vi "Connect Channels (Multiple).vi"(8 "error in (no error)":errorcluster, 10 "connection list":string, 11 "SLSC Switch in":refnum<class "SLSC Switch.lvclass">) -> (0 "error out":errorcluster, 3 "SLSC Switch out":refnum<class "SLSC Switch.lvclass">)   [LabVIEW 2015, in "SLSC Switch.lvlib" / "SLSC Switch.lvclass"]
doc: "Creates the connections between channels specified in connection list. Specify connections with two endpoints only or the explicit path between two endpoints. SLSC-SWITCH calculates and uses the shortest path between the channels. Refer to Setting Source and Configuration Channels for information about channel usage types. In the event of an error, connecting stops at the point in the list where the error occurred."
uses:
  SLSC Switch.lvclass
  slscsl/slscsl.lvclass
  <vilib>/SLSC/SLSC.lvlib
  <vilib>/SLSC/Unflatten Names (String).vi
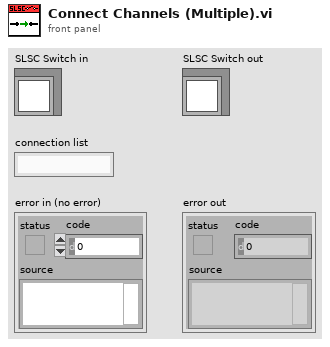
[diagram p1: front panel]
types:
  T1 = typedef "SLSC Switch.lvlib/slscsl.lvclass/SwitchActionsArray.ctl" = T2[]
  T2 = typedef "SLSC Switch.lvlib/slscsl.lvclass/SwitchAction.ctl" = cluster{"index":i32, "RelayAction":T3}
  T3 = typedef "SLSC Switch.lvlib/slscsl.lvclass/RelayAction.ctl" = u32
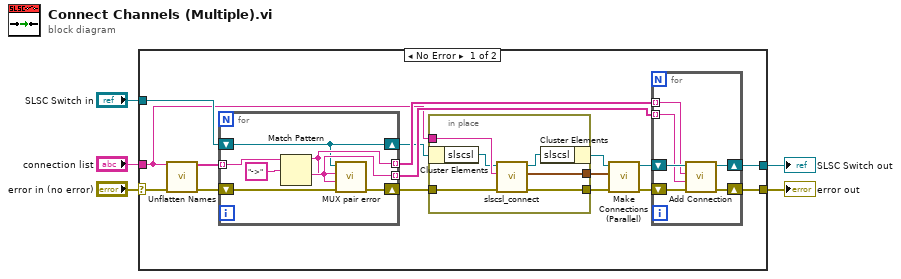
[diagram p0: block diagram]
diagram:
  n1 = case shown="No Error" "error in (no error)" {
    selector: "error in (no error)" -> [w7 w42]
    tunnel: [w13 w42] -> w2
    tunnel: [w14 w41] -> w1
    tunnel: "SLSC Switch in" -> [w18 w41]
    tunnel: "connection list" -> [w9 _]
    frame No Error {
      n2 = call-poly <vilib>:"Unflatten Names.vi"("names in"=w9, "error in (no error)"=w7) -> ("names out"=w8:string[], "error out"=w6:errorcluster)  [unwired: 12 in]
      n3 = for {
        tunnel: w8 -> [w33] mode=indexing
        shift-right: [w29] -> w10
        shift-left: w18 -> [w29]
        shift-right: [w28] -> w15
        shift-left: w6 -> [w30]
        tunnel: [w31] -> w12 mode=indexing
        tunnel: [w32] -> w11 mode=indexing
        n4 = Match Pattern(string=w33, regular expression="->") -> (before substring=w31:string, after substring=w32:string)  [unwired: 1 in, 2 out]
        n5 = call "MUX pair error.vi"("error in (no error)"=w30, "channel 2"=w32, "channel 1"=w31, "SLSC Switch in"=w29) -> ("error out"=w28:errorcluster)  [unwired: 7 in]
      }
      n6 = in-place {
        in-place-border: w9 -> [w40]
        in-place-border: w15 -> [w39]
        in-place-border: [w38] -> w19
        in-place-border: [w35] -> w20
        n7 = in-place-cluster #1(w10) -> ("slscsl"=w37:refnum<class "slscsl.lvclass">)
        n8 = call "slscsl_connect.vi"("error in (no error)"=w39, "connectionList"=w40, "slscsl in"=w37) -> ("error out"=w38:errorcluster, "switchActionsArray"=w35:T1, "slscsl out"=w36:refnum<class "slscsl.lvclass">)  [unwired: 6 in]
        n9 = in-place-cluster #1("slscsl"=w36) -> (w21:refnum<class "SLSC Switch.lvclass">)
      }
      n10 = call "Make Connections (Parallel).vi"("error in (no error)"=w19, "switchActionsArray"=w20, "SLSC Switch in"=w21) -> ("error out"=w16:errorcluster, "SLSC Switch out"=w17:refnum<class "SLSC Switch.lvclass">)  [unwired: 7 in]
      n11 = for {
        shift-right: [w26] -> w14
        shift-left: w17 -> [w27]
        shift-right: [w24] -> w13
        shift-left: w16 -> [w25]
        tunnel: w12 -> [w23] mode=indexing
        tunnel: w11 -> [w22] mode=indexing
        n12 = call "Add Connection.vi"("error in (no error)"=w25, "channel 2"=w22, "channel 1"=w23, "SLSC Switch in"=w27) -> ("error out"=w24:errorcluster, "SLSC Switch out"=w26:refnum<class "SLSC Switch.lvclass">)  [unwired: 6 in]
      }
    }
    frame Error {
    }
  }
  "error out" <- w2
  "SLSC Switch out" <- w1
